vi "LV SciSDK DIGITIZER STOP.vi"(8 "error in (no error)":errorcluster, 9 "Board Handle In":T1, 10 "Digitizer Handle In":T2) -> (0 "error out":errorcluster, 1 "Board Handle Out":T1, 2 "Digitizer Handle Out":T2)   [LabVIEW 2021, in "SciSDK_Labview.lvlib"]
uses:
  SciSDK_Labview.lvlib
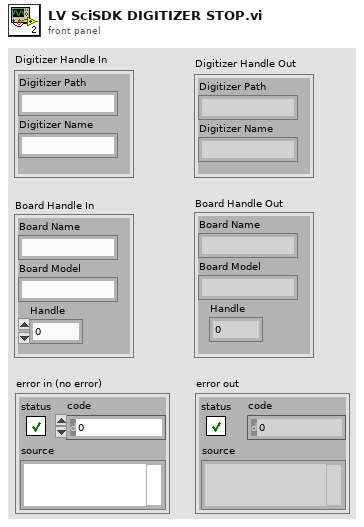
[diagram p1: front panel]
types:
  T1 = cluster{"Board Name":string, "Board Model":string, "Handle":u64}
  T2 = cluster{"Digitizer Path":string, "Digitizer Name":string}
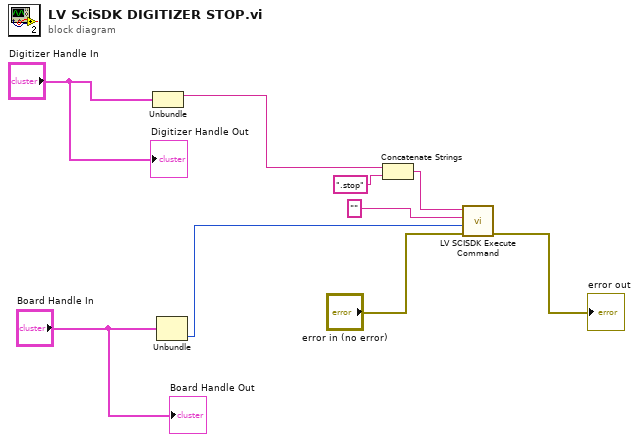
[diagram p0: block diagram]
diagram:
  n1 = Unbundle("Digitizer Handle In") -> ("Digitizer Path"=w1:string)  [unwired: 1 out]
  n2 = Unbundle("Board Handle In") -> ("Handle"=w3:u64)  [unwired: 2 out]
  n3 = Concatenate Strings(w1, ".stop" ("string")) -> (w7:string)
  n4 = call "LV SCISDK Execute Command.vi"("error in (no error)"="error in (no error)", "handle"=w3, "value"="", "Path"=w7) -> ("error out"=→"error out":errorcluster)  [unwired: 5 in, 2 out]
  "Digitizer Handle Out" <- "Digitizer Handle In"
  "Board Handle Out" <- "Board Handle In"
